vi "format set font scheme.vi"(8 "error in (no error)":errorcluster, 10 "font_scheme":string, 11 "format":u32) -> (0 "error out":errorcluster)   [LabVIEW 8.6]
doc: "void format_set_font_scheme(lxw_format format, const char *font_scheme);"
uses:
  pending_lvxlsxwriter/xlsxwriter.dll
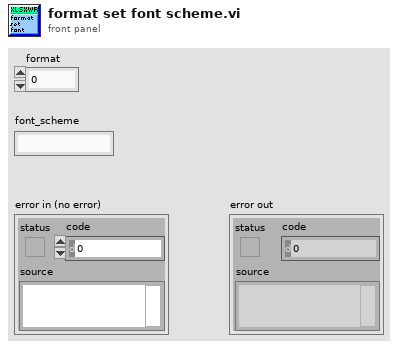
[diagram p1: front panel]
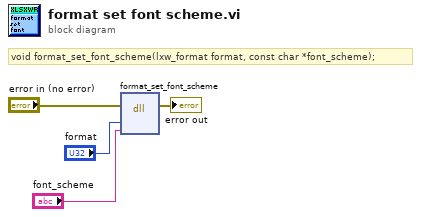
[diagram p0: block diagram]
diagram:
  # "void format_set_font_scheme(lxw_format format, const char *font_scheme);"
  n1 = dll-call lib="C:/Users/WDAGUtilityAccount/Desktop/pending_lvxlsxwriter/xlsxwriter.*" fn="format_set_font_scheme"(error in="error in (no error)", "format"="format", "font_scheme"="font_scheme") -> (error out=→"error out":errorcluster)  [unwired: 5 in, 1 out]
